vi "KE6514.ProcPeriodic.vi"(0 "i ref in":refnum<vi>, 3 "ms timeout (10000)":i32=10000, 5 "error in (no error)":errorcluster) -> (14 "i ref out":refnum<vi>, 17 "timed out":bool, 19 "error out":errorcluster)   [LabVIEW 2014, in "KE6514.lvlib"]
doc: "This method serves to periodically do things like reading values from the HW. Methods that should be executed periodically should be called from THIS methode. Add code here."
uses:
  KE6514.lvlib
  CSlibraries-extern/DimLVEvent/LVDimInterface/LVDimInterface.lvlib
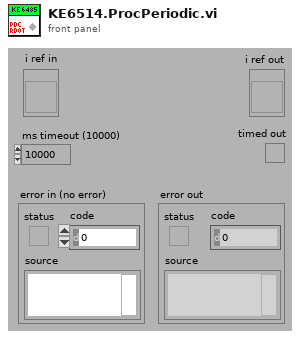
[diagram p1: front panel]
types:
  T1 = typedef "KE6514.lvlib/KE6514.i attribute.ctl" = cluster{"VISA resource name":refnum<visa-resource-name>, "ValueID":i32, "MeasurementRunning?":bool, "actSequencer":string, "actScanner":string, "actPPG":string, "MeasuredID":i32}
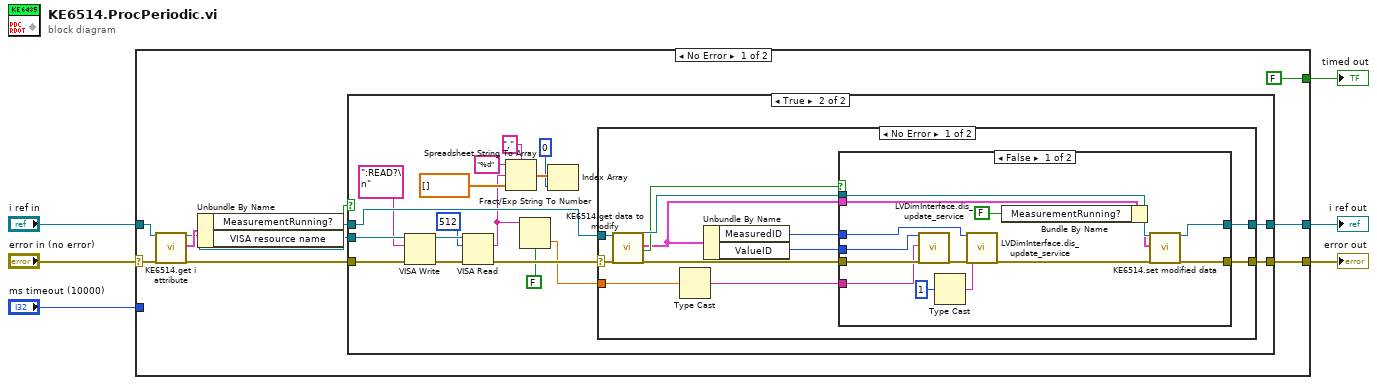
[diagram p0: block diagram]
diagram:
  n1 = case shown="No Error" "error in (no error)" {
    selector: "error in (no error)" -> [w14 w67]
    tunnel: [w8 w67] -> w5
    tunnel: "i ref in" -> [w15 w68]
    tunnel: [w10 w68] -> w3
    tunnel: [FALSE _] -> w2
    tunnel: "ms timeout (10000)" -> [_ _]
    frame No Error {
      n2 = call "KE6514.get i attribute.vi"("i ref in"=w15, "error in (no error)"=w14) -> ("i ref out"=w11:refnum<vi>, "i attribute"=w13:T1, "error out"=w9:errorcluster)  [unwired: 15 in]
      n3 = Unbundle By Name(w13) -> ("MeasurementRunning?"=w12:bool, "VISA resource name"=w7:refnum<visa-resource-name>)
      n4 = case shown="True" w12 {
        tunnel: w11 -> [w18 w35]
        tunnel: [w18 w34] -> w10
        tunnel: w9 -> [w17 w30]
        tunnel: [w17 w36] -> w8
        tunnel: w7 -> [_ w31]
        frame False {
        }
        frame True {
          n5 = VISA Write(VISA resource name=w31, write buffer=":READ?\n", error in (no error)=w30) -> (VISA resource name out=w32:refnum<visa-resource-name>, error out=w33:errorcluster)  [unwired: 1 out]
          n6 = VISA Read(VISA resource name=w32, byte count=u32 512, error in (no error)=w33) -> (read buffer=w21:string, error out=w22:errorcluster)  [unwired: 2 out]
          n7 = Spreadsheet String To Array(delimiter (Tab)=",", format string="%d", spreadsheet string=w21, array type (2D Dbl)=dbl[] []) -> (array=w24:dbl[])
          n8 = Fract/Exp String To Number(use system decimal point (T)=FALSE, string=w21) -> (number=w20:dbl)  [unwired: 2 in, 1 out]
          n9 = Index Array(array=w24, index=0) -> ()  [unwired: 1 out]
          n10 = case shown="No Error" w22 {
            selector: w22 -> [w38 w65]
            tunnel: [w48 w65] -> w36
            tunnel: w35 -> [w47 w66]
            tunnel: [w46 w66] -> w34
            tunnel: w20 -> [w39 _]
            frame No Error {
              n11 = call "KE6514.get data to modify.vi"("i ref in"=w47, "error in (no error)"=w38) -> ("i ref out"=w44:refnum<vi>, "i attribute"=w40:T1, "timed out"=w41:bool, "error out"=w45:errorcluster)  [unwired: 14 in]
              n12 = Type Cast(x=w39) -> (*(type *) &x=w42:string)  [unwired: 1 in]
              n13 = Unbundle By Name(w40) -> ("MeasuredID"=w37:i32, "ValueID"=w43:i32)
              n14 = case shown="False" w41 {
                tunnel: [w62 w64] -> w48
                tunnel: w45 -> [w61 w64]
                tunnel: w44 -> [w60 w63]
                tunnel: [w59 w63] -> w46
                tunnel: w43 -> [w58 _]
                tunnel: w42 -> [w57 _]
                tunnel: w40 -> [w56 _]
                tunnel: w37 -> [w55 _]
                frame False {
                  n15 = call "LVDimInterface.dis_update_service.vi"("my_serviceID"=w58, "data"=w57, "error in (no error)"=w61) -> ("error out"=w52:errorcluster)  [unwired: 14 in, 2 out]
                  n16 = Type Cast(x=i16 1) -> (*(type *) &x=w50:string)  [unwired: 1 in]
                  n17 = call "LVDimInterface.dis_update_service.vi"("my_serviceID"=w55, "data"=w50, "error in (no error)"=w52) -> ("error out"=w51:errorcluster)  [unwired: 14 in, 2 out]
                  n18 = Bundle By Name(cluster=w56, "MeasurementRunning?"=FALSE) -> (w54:T1)
                  n19 = call "KE6514.set modified data.vi"("i ref in"=w60, "i attribute"=w54, "error in (no error)"=w51) -> ("i ref out"=w59:refnum<vi>, "error out"=w62:errorcluster)  [unwired: 15 in]
                }
                frame True {
                }
              }
            }
            frame Error {
            }
          }
        }
      }
    }
    frame Error {
    }
  }
  "error out" <- w5
  "i ref out" <- w3
  "timed out" <- w2
